vi "Accumulate(U64).vi"(7 "enable":bool=TRUE, 8 "error in":errorcluster, 9 "reset":bool, 11 "input":u64) -> (0 "error out":errorcluster, 3 "accumulation":u64)   [LabVIEW 2012, in "Accumulate.lvlib"]
uses:
  Accumulate.lvlib
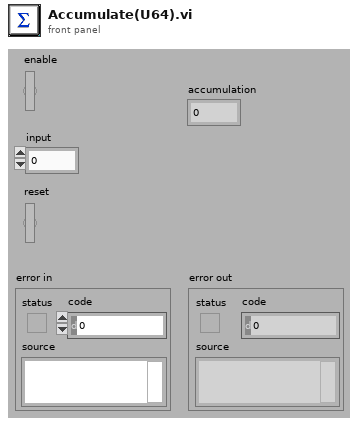
[diagram p1: front panel]
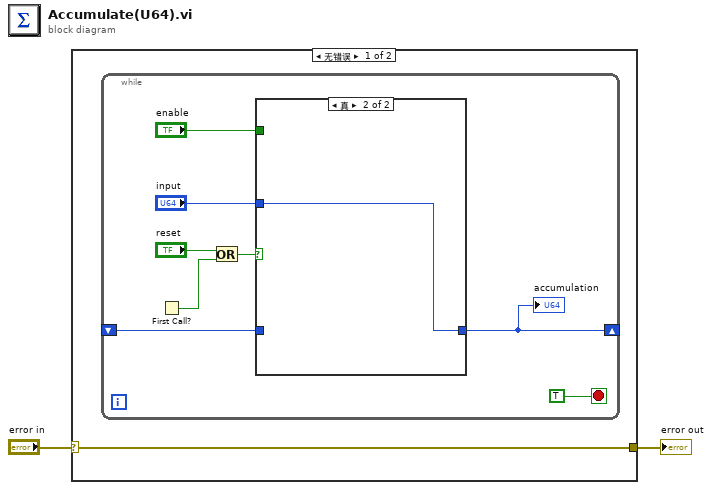
[diagram p0: block diagram]
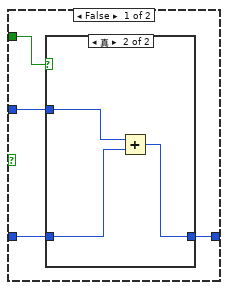
[diagram p2: hidden frame]
diagram:
  n1 = case shown="无错误" "error in" {
    selector: "error in" -> [w3 w21]
    tunnel: [w3 w21] -> w2
    frame No Error {
      n2 = while {
        shift-right: [w4] -> _
        shift-left: _ -> [w7]
        stop <- TRUE stop-if-true
        n3 = First Call?() -> (First Call?: T/F=w10:bool)
        n4 = Or(x="reset", y=w10) -> (x .or. y?=w9:bool)
        n5 = case shown="真" w9 {
          tunnel: [w12 w20] -> w4
          tunnel: "enable" -> [w15 _]
          tunnel: "input" -> [w14 w20]
          tunnel: w7 -> [w13 _]
          frame False {
            n6 = case shown="真" w15 {
              tunnel: w14 -> [_ w19]
              tunnel: w13 -> [w16 w18]
              tunnel: [w16 w17] -> w12
              frame False {
              }
              frame True {
                n7 = Add(x=w19, y=w18) -> (x+y=w17:u64)
              }
            }
          }
          frame True {
          }
        }
        "accumulation" <- w4
      }
    }
    frame Error {
    }
  }
  "error out" <- w2
